vi "analyzeAccelerationData.vi"(8 "ErrorIn":errorcluster, 11 "QueuesIn":T1) -> (0 "ErrorOut":errorcluster, 3 "QueuesOut":T1)   [LabVIEW 2019]
uses:
  utilities/Queues.ctl
  UIVIs/UIInput.ctl
  UIVIs/UIOutput.ctl
  UIVIs/AccelerationDataFrames.ctl
  communicateWebServicesVIs/WebServicesData.ctl
  analyzeAccelerationDataVIs/analyzeAccelerationDataState.ctl
  <vilib>/Waveform/WDTOps.llb/WDT Waveform Duration DBL.vi
  <vilib>/Waveform/WDTOps.llb/WDT Number of Waveform Samples DBL.vi
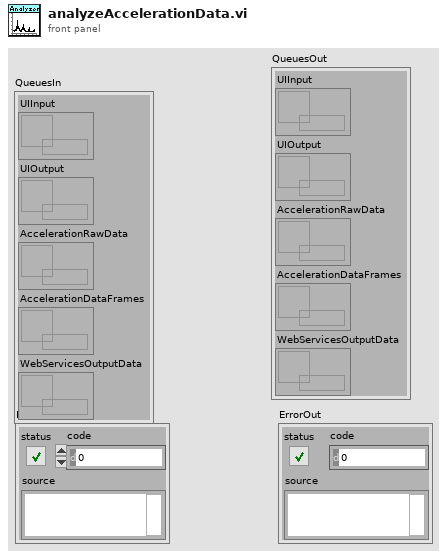
[diagram p1: front panel]
types:
  T1 = typedef "Queues.ctl" = cluster{"UIInput":refnum<queue>, "UIOutput":refnum<queue>, "AccelerationRawData":refnum<queue>, "AccelerationDataFrames":refnum<queue>, "WebServicesOutputData":refnum<queue>}
  T2 = typedef "analyzeAccelerationDataState.ctl" = enum16{"Idle", "Analyze", "Init", "EndAnalysis"}
  T3 = typedef "AccelerationDataFrames.ctl" = cluster{"AccelerationData":waveform(dbl)[], "Amplitudes":cluster{"f0":dbl, "df":dbl, "real part":dbl[]}[], "Phases":cluster{"f0":dbl, "df":dbl, "imaginary part":dbl[]}[]}
  T4 = typedef "UIInput.ctl" = cluster{"Start":bool, "Stop":bool, "Restart":bool}
  T5 = typedef "UIOutput.ctl" = cluster{"Aquiring data":bool, "CriticalError":errorcluster, "InternalError":errorcluster, "FIFO overflow":bool, "Analyzing data":bool}
  T6 = typedef "GlobalSettings.ctl" = cluster{"fs [Hz]":dbl, "Create Network Stream Timeout":i32, "Read Network Stream Timeout":i32}
  T7 = cluster{"f0":dbl, "df":dbl, "imaginary part":dbl[]}[]
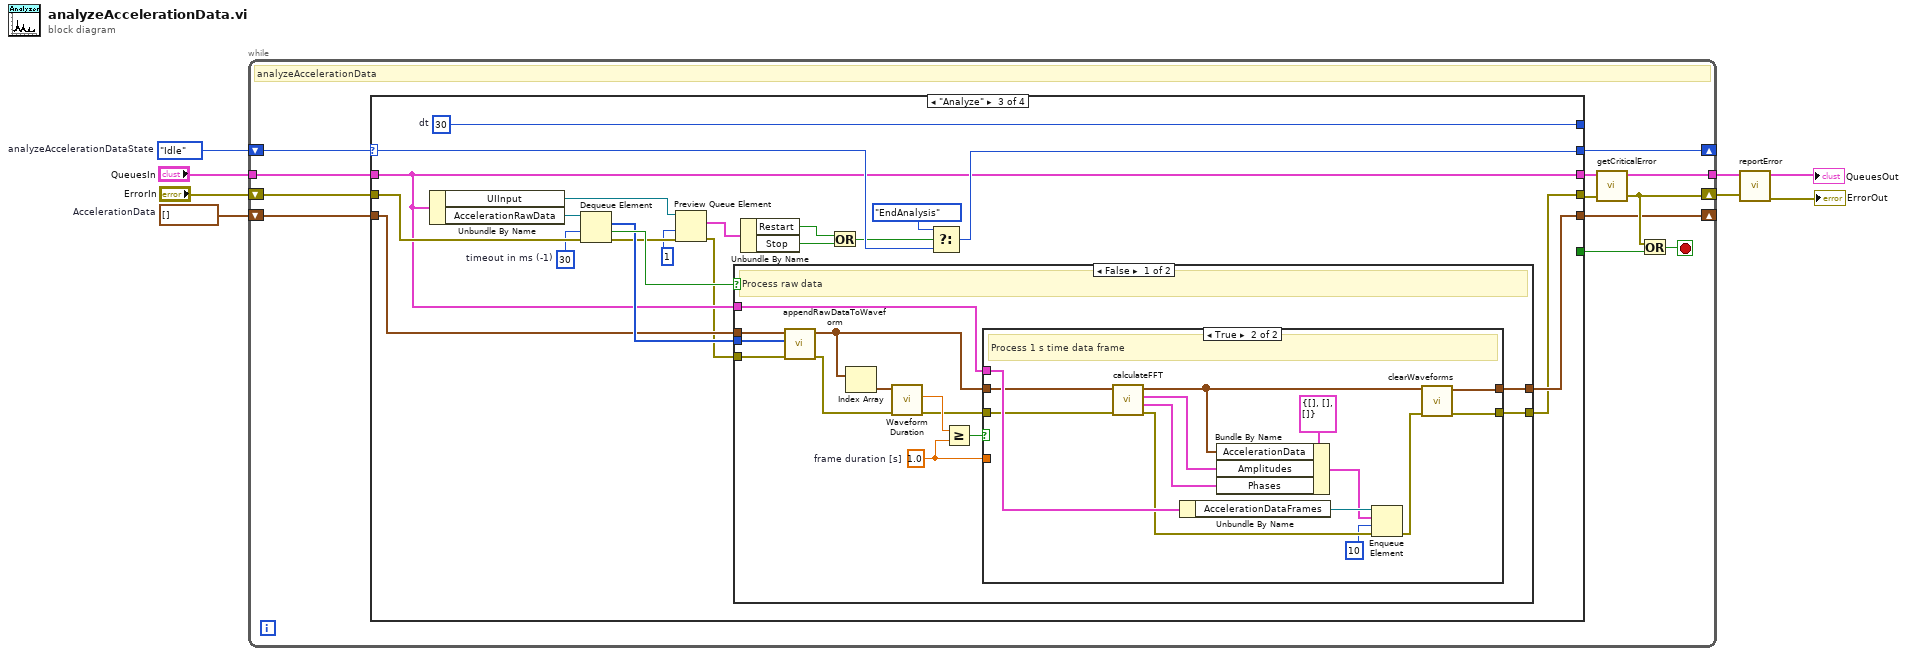
[diagram p0: block diagram]
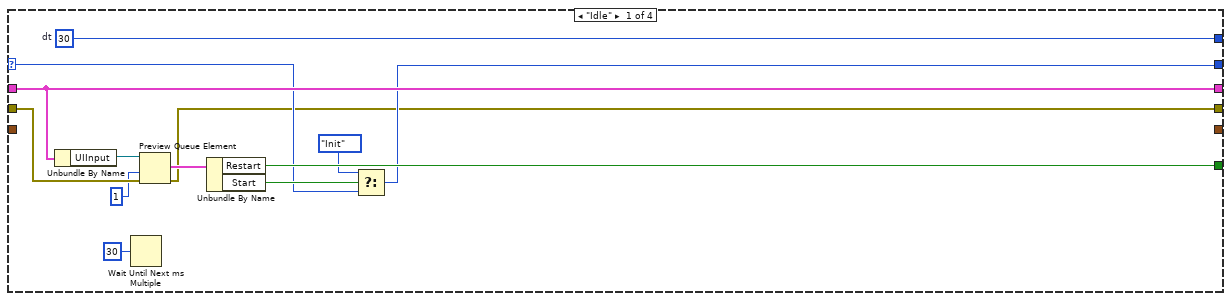
[diagram p2: hidden frame]
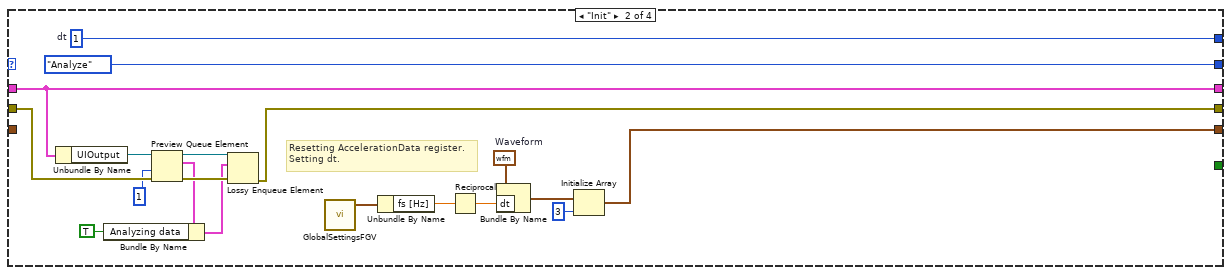
[diagram p3: hidden frame]
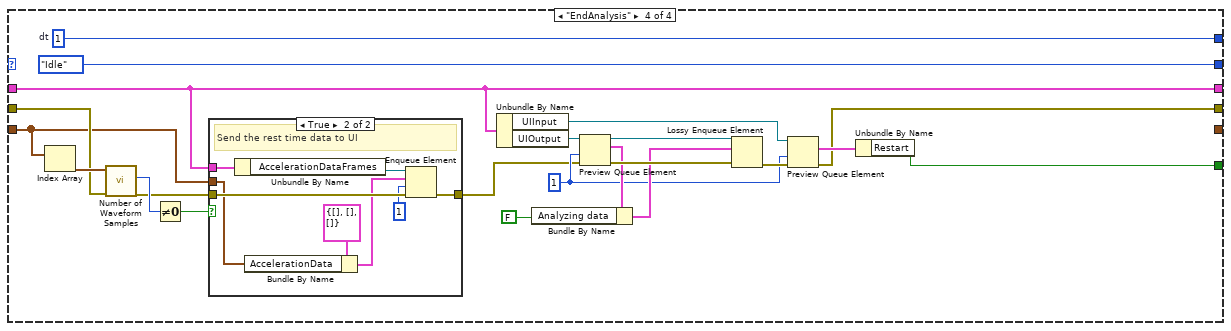
[diagram p6: hidden frame]
diagram:
  w1 = waveform(dbl)[] []  # AccelerationData
  w8 = analyzeAccelerationDataState."Idle"  # analyzeAccelerationDataState
  n1 = while {
    shift-right: [w9] -> _
    shift-left: w8 -> [w10]
    tunnel: "QueuesIn" -> [w20]
    tunnel: [w13] -> w4
    shift-right: [w14] -> w5
    shift-left: "ErrorIn" -> [w19]
    shift-right: [w11] -> _
    shift-left: w1 -> [w12]
    stop <- w17 stop-if-true
    # "analyzeAccelerationData"
    n2 = case shown="\"Analyze\"" w10 {
      selector: w10 -> [w26 _ w70 _]
      tunnel: [w24 analyzeAccelerationDataState."Analyze" ("analyzeAccelerationDataState") w66 analyzeAccelerationDataState."Idle" ("analyzeAccelerationDataState")] -> w9
      tunnel: w20 -> [w33 w43 w57 w119]
      tunnel: [w33 w43 w57 w119] -> w16
      tunnel: w19 -> [w31 w41 w73 w125]
      tunnel: [w23 w34 w55 w116] -> w15
      tunnel: [w28 _ _ w117] -> w18
      tunnel: w12 -> [_ _ w60 w123]
      tunnel: [_ w50 w59 _] -> w11
      tunnel: [w22 w49 w53 w115] -> _
      frame "Idle" {
        w22 = i64 30  # dt
        n3 = Unbundle By Name(w33) -> ("UIInput"=w32:refnum<queue>)
        n4 = Wait Until Next ms Multiple(millisecond multiple=u32 30) -> ()  [unwired: 1 out]
        n5 = Preview Queue Element(queue=w32, timeout in ms (-1)=1, error in (no error)=w31) -> (element=w29:T4, error out=w23:errorcluster)  [unwired: 2 out]
        n6 = Unbundle By Name(w29) -> ("Restart"=w28:bool, "Start"=w27:bool)
        n7 = Select(t=analyzeAccelerationDataState."Init", s=w27, f=w26) -> (s? t:f=w24:T2)
      }
      frame "Init" {
        w49 = i64 1  # dt
        w48 = waveform(dbl) {"t0"=timestamp(0 s since 1904-01-01), "dt"=0.001, "Y"=[]}  # Waveform
        # "Resetting AccelerationData register.\nSetting dt."
        n8 = Unbundle By Name(w43) -> ("UIOutput"=w42:refnum<queue>)
        n9 = Preview Queue Element(queue=w42, timeout in ms (-1)=1, error in (no error)=w41) -> (queue out=w40:refnum<queue>, element=w37:T5, error out=w39:errorcluster)  [unwired: 1 out]
        n10 = Bundle By Name(cluster=w37, "Analyzing data"=TRUE) -> (w35:T5)
        n11 = Lossy Enqueue Element(queue=w40, element=w35, error in (no error)=w39) -> (error out=w34:errorcluster)  [unwired: 3 out]
        n12 = call "GlobalSettingsFGV.vi"() -> ("GlobalSettingsOut"=w46:T6)  [unwired: 11 in]
        n13 = Unbundle By Name(w46) -> ("fs [Hz]"=w45:dbl)
        n14 = Reciprocal(x=w45) -> (1/x=w44:dbl)
        n15 = Bundle By Name(cluster=w48, "dt"=w44) -> (w47:waveform(dbl))
        n16 = Initialize Array(w47, 3 ("dimension size")) -> (w50:waveform(dbl)[])
      }
      frame "Analyze" {
        w53 = i64 30  # dt
        w72 = 30  # timeout in ms (-1)
        n17 = Unbundle By Name(w57) -> ("UIInput"=w62:refnum<queue>, "AccelerationRawData"=w61:refnum<queue>)
        n18 = Dequeue Element(queue=w61, timeout in ms (-1)=w72, error in (no error)=w73) -> (element=w64:u8[], timed out?=w65:bool, error out=w63:errorcluster)  [unwired: 1 out]
        n19 = Preview Queue Element(queue=w62, timeout in ms (-1)=1, error in (no error)=w63) -> (element=w71:T4, error out=w56:errorcluster)  [unwired: 2 out]
        n20 = case shown="False" w65 {
          tunnel: w64 -> [w85 _]
          tunnel: w56 -> [w86 w103]
          tunnel: w60 -> [w84 w104]
          tunnel: [w75 w104] -> w59
          tunnel: w57 -> [w79 _]
          tunnel: [w76 w103] -> w55
          frame False {
            w74 = 1.0  # frame duration [s]
            # "Process raw data"
            n21 = call "appendRawDataToWaveform.vi"("ErrorIn"=w86, "AccelerationRawData"=w85, "AccelerationDataIn"=w84) -> ("ErrorOut"=w83:errorcluster, "AccelerationDataOut"=w77:waveform(dbl)[])  [unwired: 7 in]
            n22 = Index Array(array=w77) -> (element=w82:waveform(dbl))  [unwired: 1 in]
            n23 = call-poly <vilib>:"Waveform Duration.vi"("error in (no error)"=w83, "waveform in"=w82) -> ("error out"=w78:errorcluster, "duration"=w81:dbl)  [unwired: 7 in, 1 out]
            n24 = Greater Or Equal?(x=w81, y=w74) -> (x >= y?=w80:bool)
            n25 = case shown="True" w80 {
              tunnel: w79 -> [_ w102]
              tunnel: w78 -> [w88 w93]
              tunnel: w77 -> [w87 w94]
              tunnel: [w88 w91] -> w76
              tunnel: [w87 w92] -> w75
              tunnel: w74 -> [_ _]
              frame False {
              }
              frame True {
                # "Process 1 s time data frame"
                n26 = call "calculateFFT.vi"("ErrorIn"=w93, "AccelerationDataIn"=w94) -> ("ErrorOut"=w101:errorcluster, "Phases"=w98:T7, "Amplitudes"=w97:cluster{"f0":dbl, "df":dbl, "real part":dbl[]}[], "AccelerationDataOut"=w90:waveform(dbl)[])  [unwired: 6 in]
                n27 = Unbundle By Name(w102) -> ("AccelerationDataFrames"=w96:refnum<queue>)
                n28 = Bundle By Name(cluster=T3 {"AccelerationData"=[], "Amplitudes"=[], "Phases"=[]} ("AccelerationDataFrames"), "AccelerationData"=w90, "Amplitudes"=w97, "Phases"=w98) -> (w95:T3)
                n29 = Enqueue Element(queue=w96, element=w95, timeout in ms (-1)=10, error in (no error)=w101) -> (error out=w89:errorcluster)  [unwired: 2 out]
                n30 = call "clearWaveforms.vi"("ErrorIn"=w89, "AccelerationDataIn"=w90) -> ("ErrorOut"=w91:errorcluster, "AccelerationDataOut"=w92:waveform(dbl)[])  [unwired: 8 in]
              }
            }
          }
          frame True {
            # "No data"
          }
        }
        n31 = Unbundle By Name(w71) -> ("Restart"=w54:bool, "Stop"=w69:bool)
        n32 = Or(x=w54, y=w69) -> (x .or. y?=w68:bool)
        n33 = Select(t=analyzeAccelerationDataState."EndAnalysis", s=w68, f=w70) -> (s? t:f=w66:T2)
      }
      frame "EndAnalysis" {
        w106 = 1 ("timeout in ms (-1)")
        w115 = i64 1  # dt
        n34 = Index Array(array=w123) -> (element=w126:waveform(dbl))  [unwired: 1 in]
        n35 = call-poly <vilib>:"Number of Waveform Samples.vi"("error in (no error)"=w125, "waveform in"=w126) -> ("error out"=w122:errorcluster, "number of samples"=w124:i32)  [unwired: 7 in, 1 out]
        n36 = Not Equal To 0?(x=w124) -> (x != 0?=w121:bool)
        n37 = case shown="True" w121 {
          tunnel: w119 -> [_ w135]
          tunnel: w122 -> [w127 w133]
          tunnel: w123 -> [_ w129]
          tunnel: [w127 w131] -> w105
          frame False {
          }
          frame True {
            # "Send the rest time data to UI"
            n38 = Unbundle By Name(w135) -> ("AccelerationDataFrames"=w134:refnum<queue>)
            n39 = Bundle By Name(cluster=T3 {"AccelerationData"=[], "Amplitudes"=[], "Phases"=[]} ("AccelerationDataFrames"), "AccelerationData"=w129) -> (w128:T3)
            n40 = Enqueue Element(queue=w134, element=w128, timeout in ms (-1)=1, error in (no error)=w133) -> (error out=w131:errorcluster)  [unwired: 2 out]
          }
        }
        n41 = Unbundle By Name(w119) -> ("UIInput"=w114:refnum<queue>, "UIOutput"=w108:refnum<queue>)
        n42 = Preview Queue Element(queue=w108, timeout in ms (-1)=w106, error in (no error)=w105) -> (queue out=w113:refnum<queue>, element=w111:T5, error out=w112:errorcluster)  [unwired: 1 out]
        n43 = Bundle By Name(cluster=w111, "Analyzing data"=FALSE) -> (w109:T5)
        n44 = Lossy Enqueue Element(queue=w113, element=w109, error in (no error)=w112) -> (error out=w107:errorcluster)  [unwired: 3 out]
        n45 = Preview Queue Element(queue=w114, timeout in ms (-1)=w106, error in (no error)=w107) -> (element=w118:T4, error out=w116:errorcluster)  [unwired: 2 out]
        n46 = Unbundle By Name(w118) -> ("Restart"=w117:bool)
      }
    }
    n47 = call "getCriticalError.vi"("ErrorIn"=w15, "QueuesIn"=w16) -> ("ErrorOut"=w14:errorcluster, "QueuesOut"=w13:T1)  [unwired: 8 in]
    n48 = Or(x=w14, y=w18) -> (x .or. y?=w17:bool)
  }
  n49 = call "reportError.vi"("ErrorIn"=w5, "QueuesIn"=w4) -> ("ErrorOut"=→"ErrorOut":errorcluster, "QueuesOut"=→"QueuesOut":T1)  [unwired: 8 in]
